vi "Read DIP Switches.vi"(8 "error in (no error)":errorcluster, 11 "GE 5565PIORC in":refnum<class "GE 5565PIORC Old.lvclass">) -> (0 "error out":errorcluster, 2 "S1":T1, 3 "GE 5565PIORC out":refnum<class "GE 5565PIORC Old.lvclass">)   [LabVIEW 2016, in "GE 5565PIORC Old.lvclass"]
uses:
  GE 5565PIORC Old.lvclass
  Controls/S1 Switch.ctl
  GE 5565PIORC Old.lvclass/GE 5565PIORC Old.ctl
  Binary Operations/Get Bits.vi
  Binary Operations/Get Bits U32.vi
  Registers/RFM Control and Status.Get Register Offset.vi
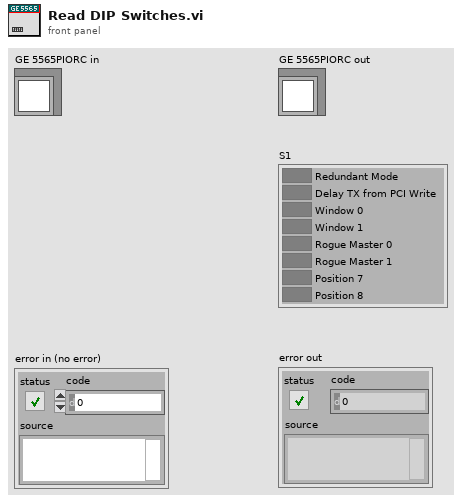
[diagram p1: front panel]
types:
  T1 = typedef "GE 5565PIORC Old.lvclass/S1 Switch.ctl" = cluster{"Redundant Mode":bool, "Delay TX from PCI Write":bool, "Window 0":bool, "Window 1":bool, "Rogue Master 0":bool, "Rogue Master 1":bool, "Position 7":bool, "Position 8":bool}
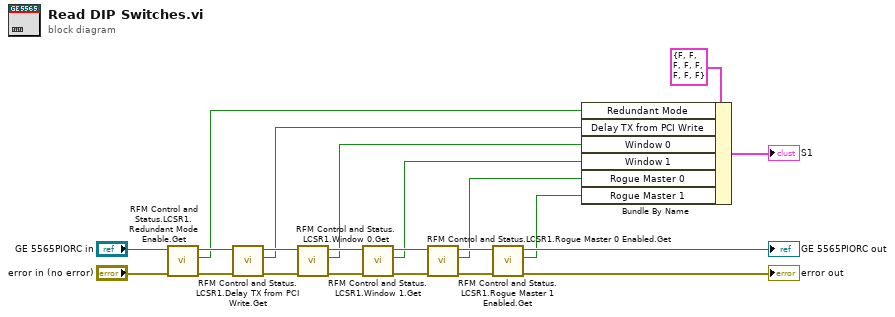
[diagram p0: block diagram]
diagram:
  n1 = call "RFM Control and Status.LCSR1.Redundant Mode Enable.Get.vi"("error in (no error)"="error in (no error)", "GE 5565PIORC"="GE 5565PIORC in") -> ("error out"=w10:errorcluster, "Redundant Mode Enabled?"=w7:bool, "GE 5565PIORC out"=w11:refnum<class "GE 5565PIORC Old.lvclass">)  [unwired: 7 in]
  n2 = call "RFM Control and Status.LCSR1.Delay TX from PCI Write.Get.vi"("error in (no error)"=w10, "GE 5565PIORC"=w11) -> ("error out"=w8:errorcluster, "Delay TX from PCI Write Enabled?"=w6:bool, "GE 5565PIORC out"=w9:refnum<class "GE 5565PIORC Old.lvclass">)  [unwired: 7 in]
  n3 = call "RFM Control and Status.LCSR1.Window 0.Get.vi"("error in (no error)"=w8, "GE 5565PIORC"=w9) -> ("error out"=w16:errorcluster, "Window 0 State"=w5:bool, "GE 5565PIORC out"=w19:refnum<class "GE 5565PIORC Old.lvclass">)  [unwired: 7 in]
  n4 = call "RFM Control and Status.LCSR1.Window 1.Get.vi"("error in (no error)"=w16, "GE 5565PIORC"=w19) -> ("error out"=w15:errorcluster, "Window 1 State"=w4:bool, "GE 5565PIORC out"=w18:refnum<class "GE 5565PIORC Old.lvclass">)  [unwired: 7 in]
  n5 = call "RFM Control and Status.LCSR1.Rogue Master 0 Enabled.Get.vi"("error in (no error)"=w15, "GE 5565PIORC"=w18) -> ("error out"=w14:errorcluster, "Rogue Master 0 Enabled?"=w3:bool, "GE 5565PIORC out"=w17:refnum<class "GE 5565PIORC Old.lvclass">)  [unwired: 7 in]
  n6 = call "RFM Control and Status.LCSR1.Rogue Master 1 Enabled.Get.vi"("error in (no error)"=w14, "GE 5565PIORC"=w17) -> ("error out"=→"error out":errorcluster, "Rogue Master 1 Enabled?"=w2:bool, "GE 5565PIORC out"=→"GE 5565PIORC out":refnum<class "GE 5565PIORC Old.lvclass">)  [unwired: 7 in]
  n7 = Bundle By Name(cluster=T1 {"Redundant Mode"=FALSE, "Delay TX from PCI Write"=FALSE, "Window 0"=FALSE, "Window 1"=FALSE, "Rogue Master 0"=FALSE, "Rogue Master 1"=FALSE, "Position 7"=FALSE, "Position 8"=FALSE} ("S1 Switch"), "Redundant Mode"=w7, "Delay TX from PCI Write"=w6, "Window 0"=w5, "Window 1"=w4, "Rogue Master 0"=w3, "Rogue Master 1"=w2) -> (→"S1":T1)
